vi "test Remove Only Alias In List.vi"(8 "error in (no error)":errorcluster, 11 "TestCase in":refnum<class "Routing and Faulting Aliases Unit Tests.lvclass">) -> (0 "error out":errorcluster, 3 "TestCase out":refnum<class "Routing and Faulting Aliases Unit Tests.lvclass">)   [LabVIEW 2020, in "Routing and Faulting Aliases Unit Tests.lvclass"]
uses:
  Routing and Faulting Aliases Unit Tests.lvclass
  System Explorer/Alias.ctl
  System Explorer/Endpoint.ctl
  Shared/Alias Endpoint.ctl
  Routing and Faulting Aliases Unit Tests.lvclass/Routing and Faulting Aliases Unit Tests.ctl
  <vilib>/addons/_JKI Toolkits/VI Tester/TestCase.llb/TestCase.lvclass
  System Explorer/Routing and Faulting System Explorer.lvlib
  Scripting/Routing and Faulting Scripting.lvlib
  Shared/Routing and Faulting Shared.lvlib
  C:/Program Files (x86)/National Instruments/LabVIEW 2020/vi.lib/addons/_JKI Toolkits/VI Tester/TestCase.llb/TestCase.lvclass
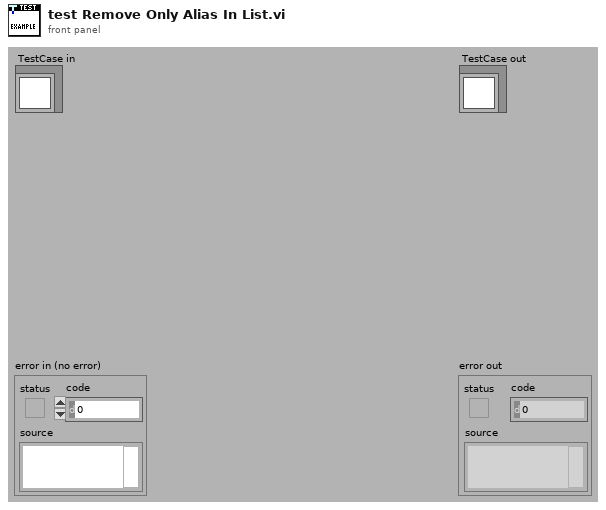
[diagram p1: front panel]
types:
  T1 = typedef "Routing and Faulting System Explorer.lvlib/Endpoint.ctl" = string
  T2 = typedef "Routing and Faulting Shared.lvlib/Alias Endpoint.ctl" = cluster{"Module Path":string, "Endpoint":string}
  T3 = typedef "Routing and Faulting System Explorer.lvlib/Alias.ctl" = cluster{"Endpoint":T1, "Alias":string, "Remove":bool}
  T4 = typedef "Custom Device API.lvlib/Custom Device Item Ref.ctl" = u64
  T5 = typedef "Routing and Faulting Shared.lvlib/Alias Mapping.ctl" = cluster{"Alias":string, "Endpoint":T2}
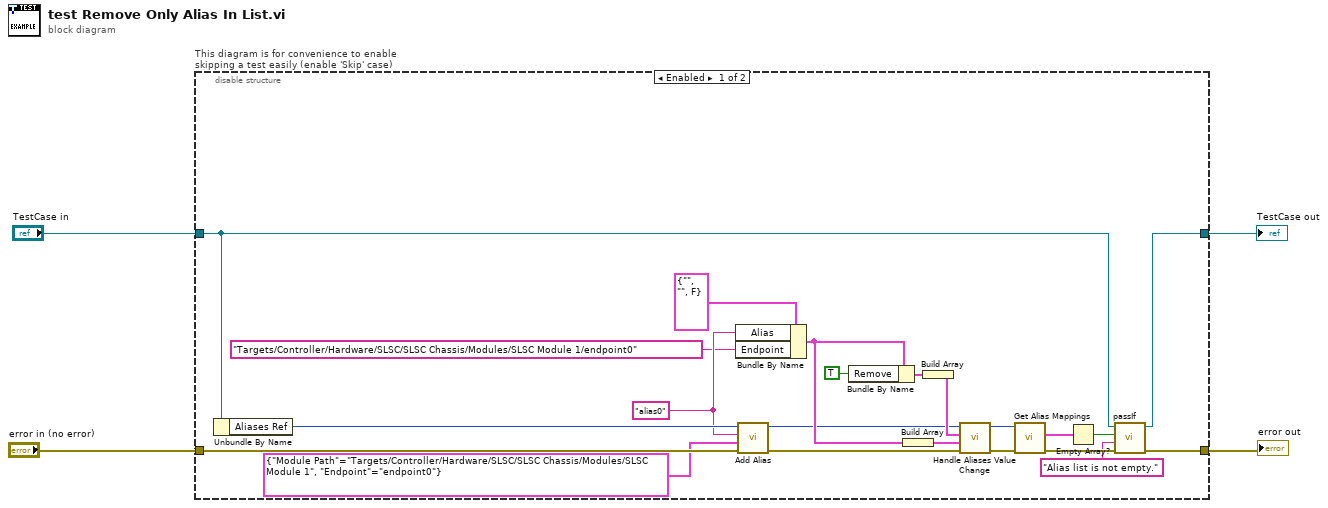
[diagram p0: block diagram]
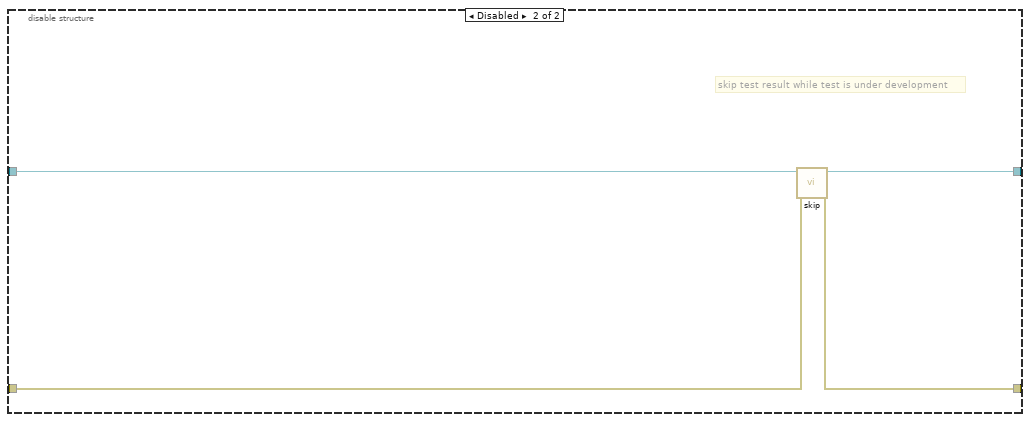
[diagram p2: hidden frame]
diagram:
  n1 = disable-structure "This diagram is for convenience to enable skipping a test easily (enable 'Skip' case)" shown="Enabled" {
    disable-tunnel: "TestCase in" -> [w22 w30]
    disable-tunnel: [w21 w28] -> w1
    disable-tunnel: [w23 w29] -> w3
    disable-tunnel: "error in (no error)" -> [w20 w27]
    frame Enabled {
      w16 = "alias0" ("Alias")
      n2 = Unbundle By Name(w22) -> ("Aliases Ref"=w19:T4)
      n3 = Bundle By Name(cluster=T3 {"Endpoint"="", "Alias"="", "Remove"=FALSE} ("Alias"), "Alias"=w16, "Endpoint"=T1 "Targets/Controller/Hardware/SLSC/SLSC Chassis/Modules/SLSC Module 1/endpoint0") -> (w12:T3)
      n4 = call "Add Alias.vi"("error in"=w20, "endpoint"=T2 {"Module Path"="Targets/Controller/Hardware/SLSC/SLSC Chassis/Modules/SLSC Module 1", "Endpoint"="endpoint0"} ("Endpoint"), "alias"=w16, "endpoint aliases in"=w19) -> ("error out"=w18:errorcluster, "endpoint aliases out"=w7:T4)  [unwired: 6 in]
      n5 = Bundle By Name(cluster=w12, "Remove"=TRUE) -> (w14:T3)
      n6 = Build Array(w12) -> (w11:T3[])
      n7 = Build Array(w14) -> (w13:T3[])
      n8 = call "Handle Aliases Value Change.vi"("error in (no error)"=w18, "OldVal"=w11, "NewVal"=w13, "Aliases Ref in"=w7) -> ("error out"=w26:errorcluster, "Aliases Ref out"=w25:T4)  [unwired: 4 in, 2 out]
      n9 = call "Get Alias Mappings.vi"("error in"=w26, "endpoint aliases in"=w25) -> ("error out"=w24:errorcluster, "alias mappings"=w10:T5[])  [unwired: 7 in, 1 out]
      n10 = Empty Array?(array=w10) -> (empty?=w9:bool)
      n11 = call-dynamic "passIf.vi"("error in (no error)"=w24, "message (\"\")"="Alias list is not empty." ("message (\"\")"), "pass"=w9, "TestCase in"=w22) -> ("error out"=w23:errorcluster, "TestCase out"=w21:refnum<class "Routing and Faulting Aliases Unit Tests.lvclass">)  [unwired: 6 in]
    }
    frame Disabled {
      # "skip test result while test is under development"
      n12 = call <vilib>:"skip.vi"("error in (no error)"=w27, "TestCase in"=w30) -> ("error out"=w29:errorcluster, "TestCase out"=w28:refnum<class "Routing and Faulting Aliases Unit Tests.lvclass">)  [unwired: 8 in]
    }
  }
  "error out" <- w3
  "TestCase out" <- w1
